vi "Viewer Control - Remove Actor.vi"(8 "error in":errorcluster, 10 "Stop Viewer Actor":refnum<class "Message Enqueuer.lvclass">, 11 "App Data in":T1) -> (0 "error out":errorcluster, 3 "App Data out":T1)   [LabVIEW 2019]
uses:
  Typedefs/#cluster_ApplicationData.ctl
  Typedefs/Acquisition Thread/#cluster_AcqQueueData.ctl
  Typedefs/Acquisition Thread/#enum_AcquisitionTask.ctl
  Typedefs/Saving Thread/#cluster_SavingQueueData.ctl
  Typedefs/Saving Thread/#enum_SavingTask.ctl
  <vilib>/ActorFramework/Message Enqueuer/Message Enqueuer.lvclass
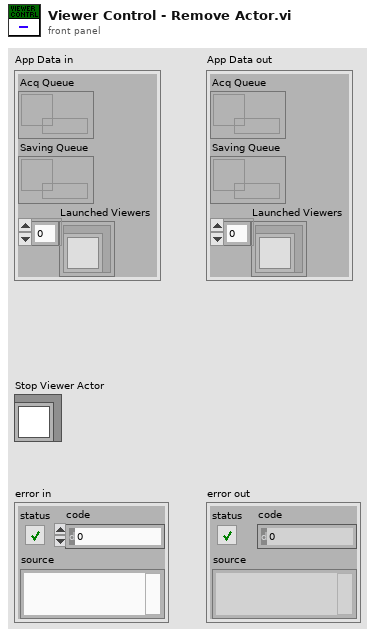
[diagram p1: front panel]
types:
  T1 = typedef "#cluster_ApplicationData.ctl" = cluster{"Acq Queue":refnum<queue>, "Saving Queue":refnum<queue>, "Launched Viewers":refnum<class "Message Enqueuer.lvclass">[]}
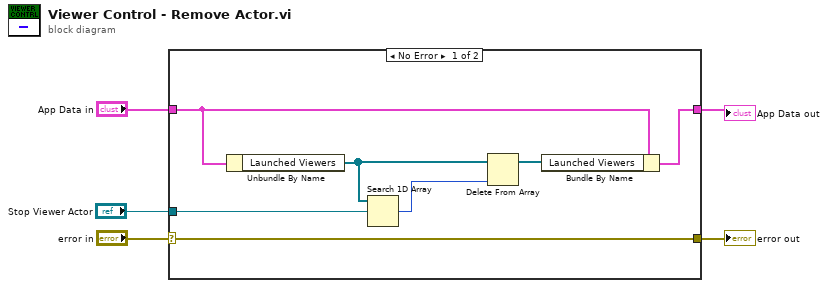
[diagram p0: block diagram]
diagram:
  n1 = case shown="No Error" "error in" {
    selector: "error in" -> [w10 w14]
    tunnel: [w12 w13] -> w5
    tunnel: "App Data in" -> [w11 w13]
    tunnel: [w10 w14] -> w2
    tunnel: "Stop Viewer Actor" -> [w9 _]
    frame No Error {
      n2 = Unbundle By Name(w11) -> ("Launched Viewers"=w8:refnum<class "Message Enqueuer.lvclass">[])
      n3 = Search 1D Array(1D array=w8, element=w9) -> (index of element=w6:i32)  [unwired: 1 in]
      n4 = Delete From Array(array=w8, index=w6) -> (array with subset deleted=w7:refnum<class "Message Enqueuer.lvclass">[])  [unwired: 1 in, 1 out]
      n5 = Bundle By Name(cluster=w11, "Launched Viewers"=w7) -> (w12:T1)
    }
    frame Error {
    }
  }
  "error out" <- w2
  "App Data out" <- w5
